vi "main.vi"() -> ()   [LabVIEW 2014]
uses:
  typedefs/ePathsAction.ctl
  typedefs/eMainAction.ctl
  typedefs/Alldata.ctl
  typedefs/NISTData.ctl
  typedefs/NIDataArray.ctl
  typedefs/NIData.ctl
  typedefs/PhasorRectangular.ctl
  typedefs/DUTData.ctl
  typedefs/NICalcAnalysis.ctl
  typedefs/CalcPhasorError.ctl
  typedefs/PlotDataArrays.ctl
  typedefs/PmuRawDataCluster.ctl
  typedefs/CalcAnalysis.ctl
  typedefs/ResultArray.ctl
  typedefs/Result.ctl
  typedefs/TVE_Fe_RFE.ctl
  <vilib>/Utility/file.llb/Write To Spreadsheet File (string).vi
panel:
  out "error out":errorcluster
  in  "btnSave":bool
  in  "btnMultiSrcAnalysis":bool
  in  "btnPlots":bool
  in  "Tab Control":T1(tab)
  out "Fluke Time":timestamp format="%^<%.3X\n%x>T"
  out "NIST Time":timestamp format="%^<%.3X\n%x>T"
  out "NIST VPhaseA Magnitude":cluster{"X":dbl, "Y":dbl}[](graph)
  out "Fluke VPhaseA Magnitude":cluster{"X":dbl, "Y":dbl}[](graph)
  out "NIST Meas - Fluke True TVE":string[][](table)
  out "NIST Meas - Fluke PMU TVE":string[][](table)
  out "CUT Results - CCS Results TVE":string[][](table)
  out "Results Table":string[][](table)
  in  "btnSrcAnalysis":bool
  in  "btnExit":bool
  in  "error in (no error)":errorcluster
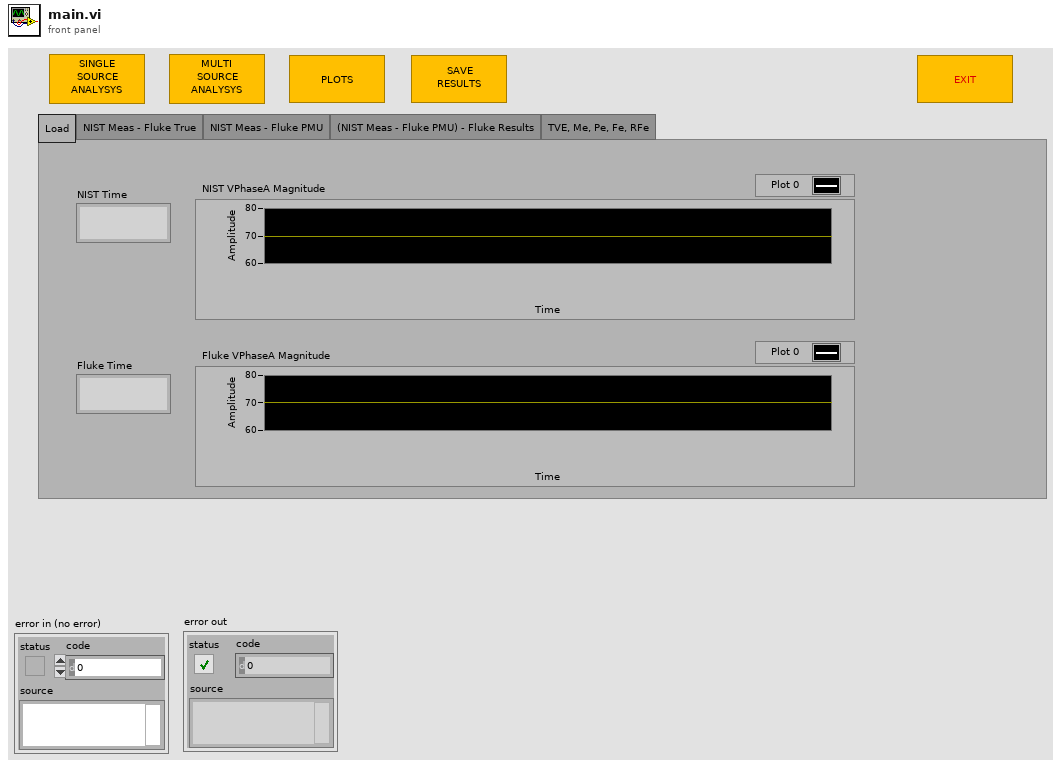
[diagram p1: front panel]
types:
  T1 = enum32{"Load", "NIST Meas - Fluke True", "NIST Meas - Fluke PMU", "(NIST Meas - Fluke PMU) - Fluke Results", "TVE, Me, Pe, Fe, RFe"}
  T2 = typedef "ResultArray.ctl" = T3[]
  T3 = typedef "Result.ctl" = cluster{"Time Stamp":timestamp, "VPhaseA":T4, "VPhaseB":T4, "VPhaseC":T4, "IPhaseA":T4, "IPhaseB":T4, "IPhaseC":T4}
  T4 = typedef "TVE_Fe_RFE.ctl" = cluster{"TVE":dbl, "Fe":dbl, "RFe":dbl}
  T5 = typedef "Alldata.ctl" = cluster{"NISTData":T6, "FlukeData":T13, "Params":dbl[]}
  T6 = typedef "NISTData.ctl" = cluster{"NIDataArray":T7, "DUTDataArray":T10[], "DataAnlysisArray":T11[]}
  T7 = typedef "NIDataArray.ctl" = T8[]
  T8 = typedef "NIData.ctl" = cluster{"Time":dbl, "VA":T9, "VB":T9, "VC":T9, "V+":T9, "IA":T9, "IB":T9, "IC":T9, "I+":T9, "Freq":dbl, "ROCOF":dbl, "TimeStamp":timestamp}
  T9 = typedef "PhasorRectangular.ctl" = cluster{"Real":dbl, "Imaginary":dbl}
  T10 = typedef "DUTData.ctl" = cluster{"Time":dbl, "VA":T9, "VB":T9, "VC":T9, "V1":T9, "IA":T9, "IB":T9, "IC":T9, "I1":T9, "Freq":dbl, "ROCOF":dbl, "TimeStamp":timestamp}
  T11 = typedef "NICalcAnalysis.ctl" = cluster{"Time":dbl, "VPhaseA":T12, "VPhaseB":T12, "VPhaseC":T12, "VPosSeq":T12, "IPhaseA":T12, "IPhaseB":T12, "IPhaseC":T12, "IPosSeq":T12, "Fe":dbl, "RFe":dbl, "TimeStamp":timestamp}
  T12 = typedef "CalcPhasorError.ctl" = cluster{"TVE":dbl, "MagErr":dbl, "PhaseErr":dbl}
  T13 = typedef "PlotDataArrays.ctl" = cluster{"PMUDataArray":T14[], "ModelDataArray":T14[], "DataAnalysisArray":T15[]}
  T14 = typedef "PmuRawDataCluster.ctl" = cluster{"TimeStamp":timestamp, "VPhaseA":T9, "VPhaseB":T9, "VPhaseC":T9, "VPosSeq":T9, "IPhaseA":T9, "IPhaseB":T9, "IPhaseC":T9, "IPosSeq":T9, "FREQUENCY":dbl, "ROCOF":sgl}
  T15 = typedef "CalcAnalysis.ctl" = cluster{"TimeStamp":timestamp, "VPhaseA":T12, "VPhaseB":T12, "VPhaseC":T12, "VPosSeq":T12, "IPhaseA":T12, "IPhaseB":T12, "IPhaseC":T12, "IPosSeq":T12, "Fe":dbl, "RFe":dbl}
  T16 = typedef "eMainAction.ctl" = enum16{"Init", "ProcessUI", "Exit"}
  T17 = typedef "ePathsAction.ctl" = enum16{"Set", "Get", "Load", "Save", "Default", "Exit"}
  T18 = enum32{"Load", "NIST Meas - Fluke True", "NIST Meas - Fluke PMU", "(NIST Meas - Fluke PMU) - Fluke Results"}
  T19 = typedef "Paths.ctl" = cluster{"BasePath":path, "CutPath":path, "LastCutPath":path, "CCSPath":path, "LastCCSPath":path, "ResultsPath":path}
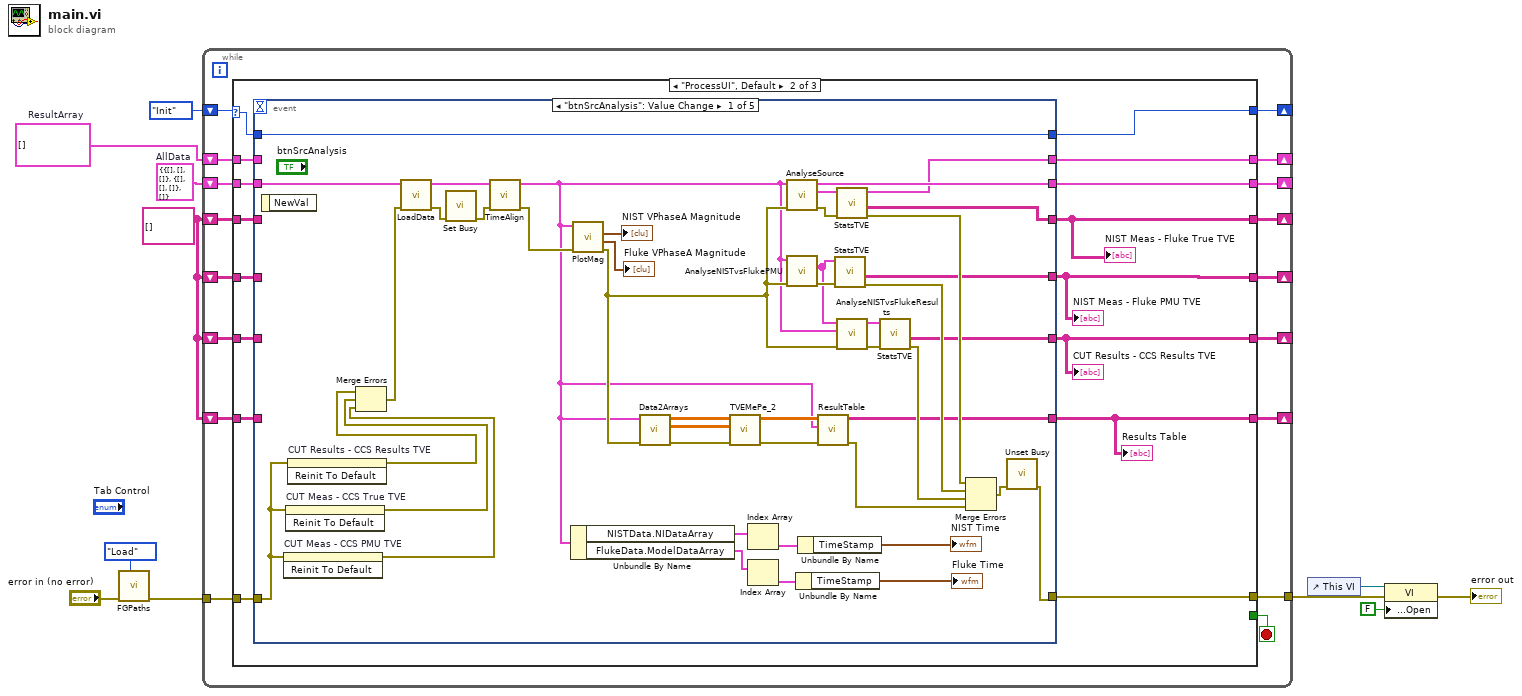
[diagram p0: block diagram]
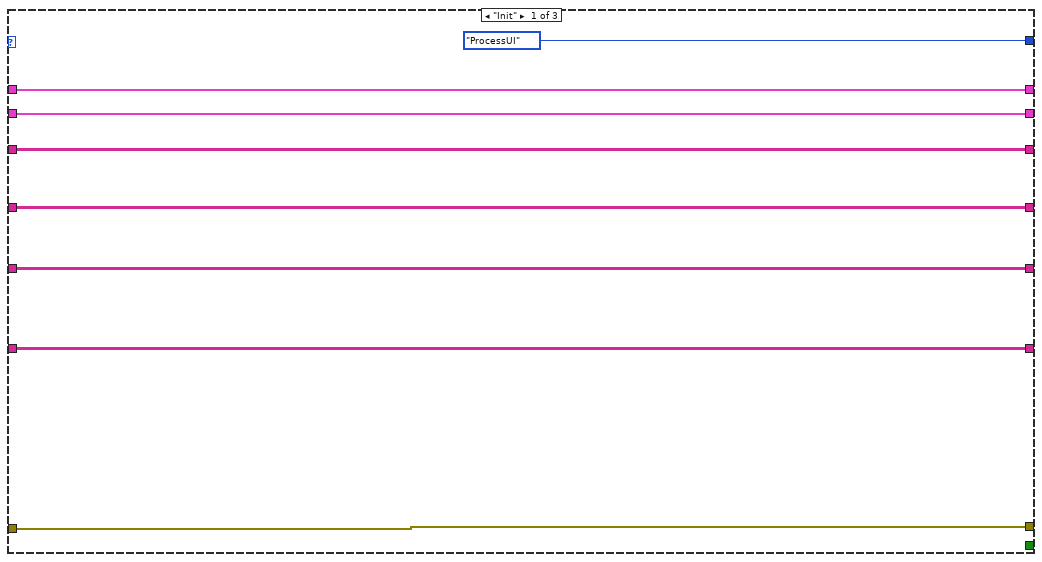
[diagram p2: hidden frame]
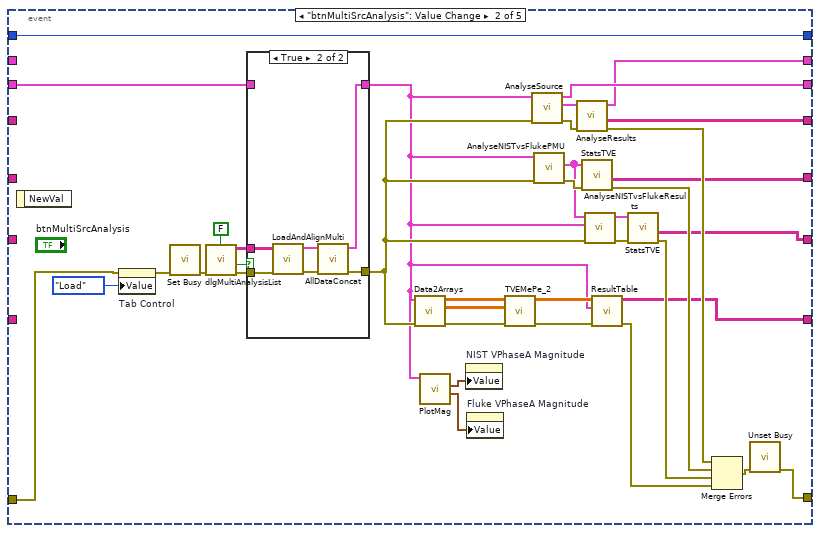
[diagram p3: hidden frame]
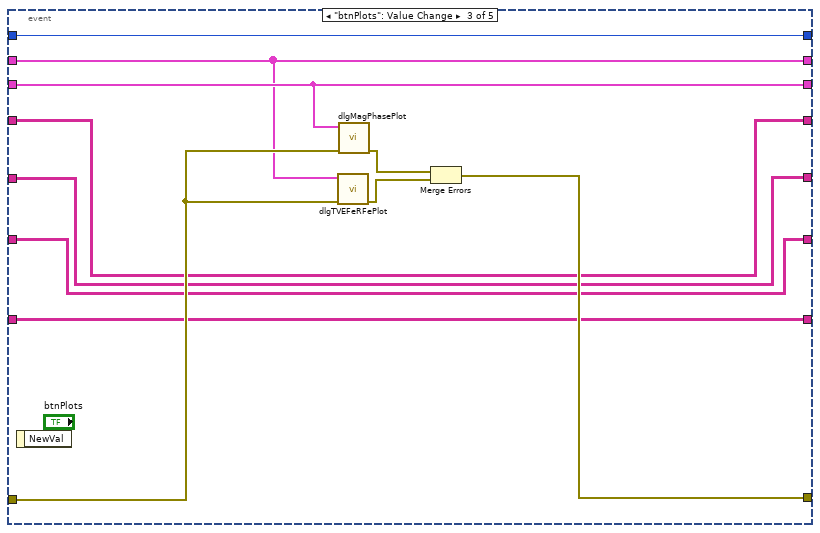
[diagram p5: hidden frame]
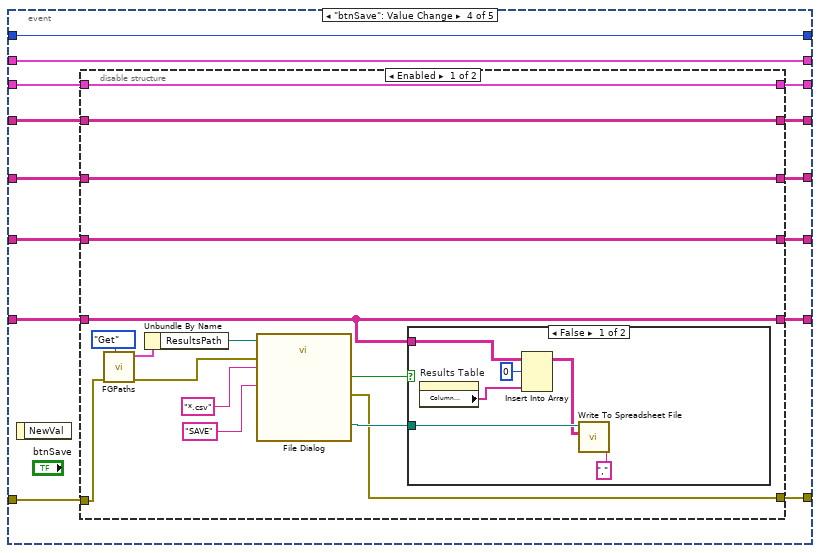
[diagram p6: hidden frame]
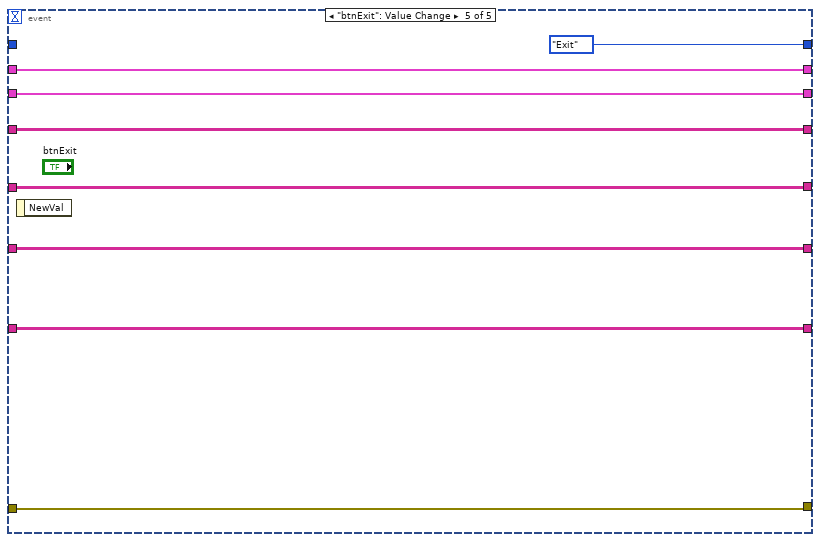
[diagram p9: hidden frame]
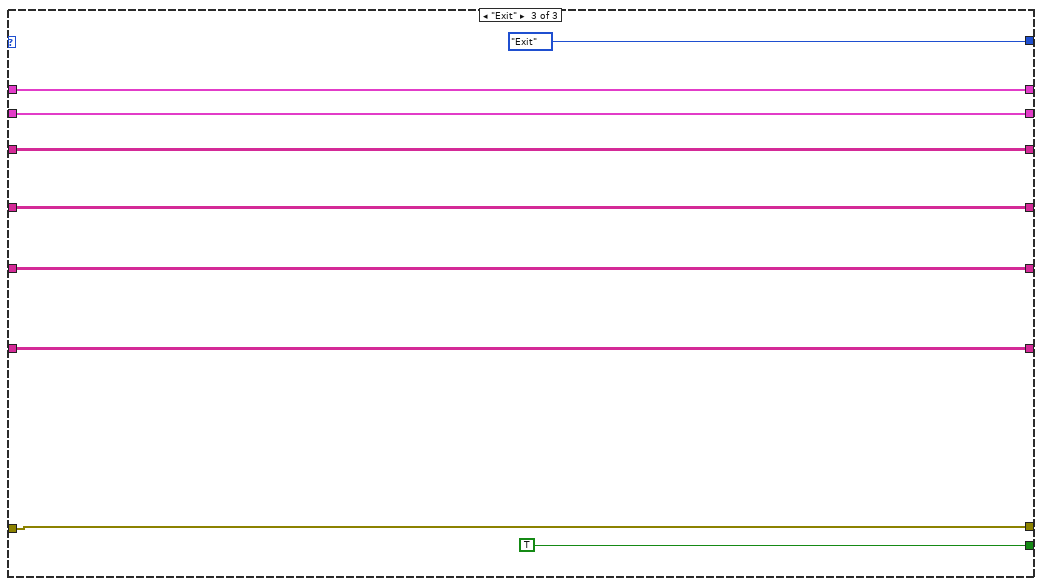
[diagram p10: hidden frame]
diagram:
  w2 = string[][] [] ("StringArray")
  w6 = T2 []  # ResultArray
  w7 = T5 {"NISTData"={"NIDataArray"=[], "DUTDataArray"=[], "DataAnlysisArray"=[]}, "FlukeData"={"PMUDataArray"=[], "ModelDataArray"=[], "DataAnalysisArray"=[]}, "Params"=[]}  # AllData
  n1 = call "FGPaths.vi"("ePathsAction"=ePathsAction."Load", "error in (no error)"="error in (no error)") -> ("error out"=w8:errorcluster)  [unwired: 8 in, 1 out]
  n2 = while {
    shift-right: [w27] -> _
    shift-left: eMainAction."Init" ("eMainAction") -> [w28]
    tunnel: w8 -> [w26]
    tunnel: [w25] -> w4
    shift-right: [w22] -> _
    shift-left: w7 -> [w23]
    shift-right: [w21] -> _
    shift-left: w6 -> [w20]
    shift-right: [w19] -> _
    shift-left: w2 -> [w18]
    shift-right: [w17] -> _
    shift-left: w2 -> [w16]
    shift-right: [w15] -> _
    shift-left: w2 -> [w14]
    shift-right: [w13] -> _
    shift-left: w2 -> [w12]
    stop <- w24 stop-if-true
    n3 = case shown="\"ProcessUI\", Default" w28 {
      selector: w28 -> [_ w49 _]
      tunnel: [eMainAction."ProcessUI" ("eMainAction") w50 eMainAction."Exit" ("eMainAction")] -> w27
      tunnel: w26 -> [w35 w52 w208]
      tunnel: [w35 w51 w208] -> w25
      tunnel: [_ _ TRUE] -> w24
      tunnel: [w34 w48 w206] -> w22
      tunnel: w23 -> [w34 w47 w206]
      tunnel: [w33 w46 w207] -> w21
      tunnel: w20 -> [w33 w45 w207]
      tunnel: [w32 w41 w205] -> w19
      tunnel: w18 -> [w32 w44 w205]
      tunnel: [w31 w43 w204] -> w17
      tunnel: w16 -> [w31 w42 w204]
      tunnel: [w30 w39 w203] -> w15
      tunnel: w14 -> [w30 w40 w203]
      tunnel: [w29 w38 w202] -> w13
      tunnel: w12 -> [w29 w37 w202]
      frame "Init" {
      }
      frame "ProcessUI", Default {
        n4 = event shown="[0] \"btnSrcAnalysis\": Value Change" {
          selector: _ -> [_ _ _ _ _]
          dyn-events: _ -> [_ _ _ _ _]
          timeout: _ -> [_ _ _ _ _]
          tunnel: [w88 w122 w147 w162 w197] -> w51
          tunnel: w52 -> [w66 w124 w151 w164 w197]
          tunnel: [w78 w121 w146 w166 eMainAction."Exit" ("eMainAction")] -> w50
          tunnel: w49 -> [w78 w121 w146 w166 _]
          tunnel: [w95 w128 w152 w160 w200] -> w48
          tunnel: w47 -> [w91 w129 w152 w161 w200]
          tunnel: [w94 w125 w150 w165 w199] -> w46
          tunnel: w45 -> [_ _ w150 w165 w199]
          tunnel: [w77 w120 w145 w155 w198] -> w41
          tunnel: w44 -> [_ _ w145 w163 w198]
          tunnel: [w72 w116 w144 w158 w196] -> w43
          tunnel: w42 -> [_ _ w144 w159 w196]
          tunnel: [w63 w109 w143 w156 w195] -> w39
          tunnel: w40 -> [_ _ w143 w157 w195]
          tunnel: [w55 w101 w142 w154 w194] -> w38
          tunnel: w37 -> [_ _ w142 w153 w194]
          event "btnSrcAnalysis": Value Change {
            n5 = event-data() -> ()  [unwired: 1 in, 1 out]
            n6 = invoke on="CUT Meas - CCS PMU TVE" class="Tbl (strict)" method="Reinit To Default"(error in=w66) -> (error out=w71:errorcluster)  [unwired: 2 in, 2 out]
            n7 = invoke on="CUT Meas - CCS True TVE" class="Tbl (strict)" method="Reinit To Default"(error in=w66) -> (error out=w70:errorcluster)  [unwired: 2 in, 2 out]
            n8 = invoke on="CUT Results - CCS Results TVE" class="Tbl (strict)" method="Reinit To Default"(error in=w66) -> (error out=w68:errorcluster)  [unwired: 2 in, 2 out]
            n9 = Merge Errors(w68, w70, w71) -> (w69:errorcluster)
            n10 = call "LoadData.vi"("error in (no error)"=w69, "AllData In"=w91) -> ("error out"=w90:errorcluster, "AllData Out"=w92:T5)  [unwired: 8 in]
            n11 = call <vilib>:"Set Busy.vi"("error in (no error)"=w90) -> ("error out"=w89:errorcluster)  [unwired: 9 in, 1 out]
            n12 = call "TimeAlign.vi"("error in (no error)"=w89, "AllData In"=w92) -> ("error out"=w87:errorcluster, "AllData Out"=w54:T5)  [unwired: 8 in]
            n13 = Unbundle By Name(w54) -> ("NISTData.NIDataArray"=w84:T7, "FlukeData.ModelDataArray"=w83:T14[])
            n14 = call "PlotMag.vi"("error in (no error)"=w87, "AllData In"=w54) -> ("error out"=w58:errorcluster, "NistPlot"=→"Fluke VPhaseA Magnitude":cluster{"X":dbl, "Y":dbl}[], "FlukePlot"=→"NIST VPhaseA Magnitude":cluster{"X":dbl, "Y":dbl}[])  [unwired: 7 in]
            n15 = call "Data2Arrays.vi"("error in (no error)"=w58, "AllData"=w54) -> ("error out"=w57:errorcluster, "Fluke"=w60:dbl[][], "NIST"=w61:dbl[][])  [unwired: 7 in]
            n16 = call "TVEMePe_2.vi"("error in (no error)"=w57, "Fluke"=w60, "NIST"=w61) -> ("error out"=w56:errorcluster, "TVEMePe"=w59:dbl[][])  [unwired: 7 in]
            n17 = Index Array(array=w84) -> (element=w82:T8)  [unwired: 1 in]
            n18 = Index Array(array=w83) -> (element=w81:T14)  [unwired: 1 in]
            n19 = call "AnalyseSource.vi"("error in (no error)"=w58, "AllData In"=w54) -> ("error out"=w93:errorcluster, "ResultArray"=w96:T2, "AllData Out"=w95:T5)  [unwired: 7 in]
            n20 = call "AnalyseNISTvsFlukePMU.vi"("error in (no error)"=w58, "AllData In"=w54) -> ("error out"=w76:errorcluster, "ResultArray"=w67:T2)  [unwired: 7 in, 1 out]
            n21 = Unbundle By Name(w81) -> ("TimeStamp"=→"Fluke Time":timestamp)
            n22 = Unbundle By Name(w82) -> ("TimeStamp"=→"NIST Time":timestamp)
            n23 = call "ResultTable.vi"("error in (no error)"=w56, "AllData"=w54, "TVEMePe"=w59) -> ("error out"=w53:errorcluster, "Results Table"=w55:string[][])  [unwired: 7 in]
            n24 = call "StatsTVE.vi"("error in (no error)"=w76, "ResultArrayIn"=w67) -> ("error out"=w73:errorcluster, "StringArray"=w72:string[][])  [unwired: 6 in, 2 out]
            n25 = call "StatsTVE.vi"("error in (no error)"=w93, "ResultArrayIn"=w96) -> ("error out"=w74:errorcluster, "StringArray"=w77:string[][], "ResultArrayOut"=w94:T2)  [unwired: 6 in, 1 out]
            n26 = call "AnalyseNISTvsFlukeResults.vi"("error in (no error)"=w58, "AllData In"=w54, "NISTResults"=w67) -> ("error out"=w65:errorcluster, "Resultarray"=w64:T3[])  [unwired: 7 in]
            n27 = call "StatsTVE.vi"("error in (no error)"=w65, "ResultArrayIn"=w64) -> ("error out"=w62:errorcluster, "StringArray"=w63:string[][])  [unwired: 6 in, 2 out]
            n28 = Merge Errors(w74, w73, w62, w53) -> (w75:errorcluster)
            n29 = call <vilib>:"Unset Busy.vi"("error in (no error)"=w75) -> ("error out"=w88:errorcluster)  [unwired: 10 in]
          }
          event "btnMultiSrcAnalysis": Value Change {
            n30 = event-data() -> ()  [unwired: 1 in, 1 out]
            n31 = property on="Tab Control" class="TabCtl (strict)"(error in=w124, "Value"=T18."Load" ("Tab Control")) -> (error out=w97:errorcluster)  [unwired: 1 in, 1 out]
            n32 = call <vilib>:"Set Busy.vi"("error in (no error)"=w97) -> ("error out"=w123:errorcluster)  [unwired: 9 in, 1 out]
            n33 = call "dlgMultiAnalysisList.vi"("StandAlone (true)"=FALSE, "error in (no error)"=w123) -> ("error out"=w131:errorcluster, "Analyse"=w132:bool, "FileList"=w130:string[][])  [unwired: 7 in]
            n34 = case shown="True" w132 {
              tunnel: w131 -> [w135 w140]
              tunnel: [w135 w136] -> w102
              tunnel: w130 -> [_ w141]
              tunnel: [w134 w138] -> w98
              tunnel: w129 -> [w134 _]
              frame False {
              }
              frame True {
                n35 = call "LoadAndAlignMulti.vi"("error in (no error)"=w140, "FileList"=w141) -> ("error out"=w137:errorcluster, "AllDataArray"=w139:T5[])  [unwired: 8 in]
                n36 = call "AllDataConcat.vi"("error in (no error)"=w137, "AllDataArray"=w139) -> ("error out"=w136:errorcluster, "AllData"=w138:T5)  [unwired: 8 in]
              }
            }
            n37 = call "Data2Arrays.vi"("error in (no error)"=w102, "AllData"=w98) -> ("error out"=w105:errorcluster, "Fluke"=w107:dbl[][], "NIST"=w108:dbl[][])  [unwired: 7 in]
            n38 = call "PlotMag.vi"("AllData In"=w98) -> ("NistPlot"=w100:cluster{"X":dbl, "Y":dbl}[], "FlukePlot"=w99:cluster{"X":dbl, "Y":dbl}[])  [unwired: 8 in, 1 out]
            n39 = property on="NIST VPhaseA Magnitude" class="XYGraph (strict)"("Value"=w99) -> ()  [unwired: 2 in, 2 out]
            n40 = property on="Fluke VPhaseA Magnitude" class="XYGraph (strict)"("Value"=w100) -> ()  [unwired: 2 in, 2 out]
            n41 = call "TVEMePe_2.vi"("error in (no error)"=w105, "Fluke"=w107, "NIST"=w108) -> ("error out"=w104:errorcluster, "TVEMePe"=w106:dbl[][])  [unwired: 7 in]
            n42 = call "AnalyseSource.vi"("error in (no error)"=w102, "AllData In"=w98) -> ("error out"=w126:errorcluster, "ResultArray"=w127:T2, "AllData Out"=w128:T5)  [unwired: 7 in]
            n43 = call "AnalyseNISTvsFlukePMU.vi"("error in (no error)"=w102, "AllData In"=w98) -> ("error out"=w117:errorcluster, "ResultArray"=w111:T2)  [unwired: 7 in, 1 out]
            n44 = call "AnalyseResults.vi"("error in (no error)"=w126, "ResultArrayIn"=w127) -> ("error out"=w118:errorcluster, "StringArray"=w120:string[][], "ResultArrayOut"=w125:T2)  [unwired: 6 in, 1 out]
            n45 = call "StatsTVE.vi"("error in (no error)"=w117, "ResultArrayIn"=w111) -> ("error out"=w115:errorcluster, "StringArray"=w116:string[][])  [unwired: 6 in, 2 out]
            n46 = call "AnalyseNISTvsFlukeResults.vi"("error in (no error)"=w102, "AllData In"=w98, "NISTResults"=w111) -> ("error out"=w113:errorcluster, "Resultarray"=w112:T3[])  [unwired: 7 in]
            n47 = call "ResultTable.vi"("error in (no error)"=w104, "AllData"=w98, "TVEMePe"=w106) -> ("error out"=w103:errorcluster, "Results Table"=w101:string[][])  [unwired: 7 in]
            n48 = call "StatsTVE.vi"("error in (no error)"=w113, "ResultArrayIn"=w112) -> ("error out"=w110:errorcluster, "StringArray"=w109:string[][])  [unwired: 6 in, 2 out]
            n49 = Merge Errors(w118, w115, w110, w103) -> (w119:errorcluster)
            n50 = call <vilib>:"Unset Busy.vi"("error in (no error)"=w119) -> ("error out"=w122:errorcluster)  [unwired: 10 in]
          }
          event "btnPlots": Value Change {
            n51 = event-data() -> ()  [unwired: 1 in, 1 out]
            n52 = call "dlgTVEFeRFePlot.vi"("error in (no error)"=w151, "ResultArray"=w150) -> ("error out"=w149:errorcluster)  [unwired: 9 in]
            n53 = call "dlgMagPhasePlot.vi"("error in (no error)"=w151, "AllData"=w152) -> ("error out"=w148:errorcluster)  [unwired: 9 in]
            n54 = Merge Errors(w148, w149) -> (w147:errorcluster)
          }
          event "btnSave": Value Change {
            n55 = event-data() -> ()  [unwired: 1 in, 1 out]
            n56 = disable-structure shown="Enabled" {
              disable-tunnel: w164 -> [w180 w189]
              disable-tunnel: w163 -> [w168 w193]
              disable-tunnel: [w176 w189] -> w162
              disable-tunnel: w161 -> [w171 w190]
              disable-tunnel: [w171 w190] -> w160
              disable-tunnel: w159 -> [w170 w192]
              disable-tunnel: [w170 w192] -> w158
              disable-tunnel: w157 -> [w169 w191]
              disable-tunnel: [w169 w191] -> w156
              disable-tunnel: [w168 w193] -> w155
              disable-tunnel: [w167 w188] -> w154
              disable-tunnel: w153 -> [w167 w188]
              frame Enabled {
                n57 = call "FGPaths.vi"("ePathsAction"=ePathsAction."Get", "error in (no error)"=w180) -> ("error out"=w177:errorcluster, "PathsOut"=w179:T19)  [unwired: 8 in]
                n58 = Unbundle By Name(w179) -> ("ResultsPath"=w175:path)
                n59 = call "File Dialog"("start path"=w175, "button label"="SAVE", "error in"=w177, "pattern (all files)"="*.csv") -> ("selected path"=w178:path, "cancelled"=w172:bool, "error out"=w176:errorcluster)  [unwired: 8 in, 1 out]
                n60 = case shown="False" w172 {
                  tunnel: w167 -> [w185 _]
                  tunnel: w178 -> [w186 _]
                  frame False {
                    n61 = property on="Results Table" class="Tbl (strict)"() -> ("Column Headers[]"=w182:string[])  [unwired: 2 in, 2 out]
                    n62 = Insert Into Array(array=w185, index (row)=0, new element=w182) -> (w183:string[][])  [unwired: 1 in]
                    n63 = call-poly <vilib>:"Write To Spreadsheet File.vi"("delimiter (\\t)"="," ("delimiter (\\t)"), "2D data"=w183, "file path (dialog if empty)"=w186) -> ()  [unwired: 5 in, 1 out]
                  }
                  frame True {
                  }
                }
              }
              frame Disabled {
              }
            }
          }
          event "btnExit": Value Change {
            n64 = event-data() -> ()  [unwired: 1 in, 1 out]
          }
        }
        "NIST Meas - Fluke PMU TVE" <- w43
        "NIST Meas - Fluke True TVE" <- w41
        "CUT Results - CCS Results TVE" <- w39
        "Results Table" <- w38
      }
      frame "Exit" {
      }
    }
  }
  n65 = control-ref of="This VI"() -> (w5:refnum<vi>)
  n66 = property class="VI"(reference=w5, error in=w4, "Front Panel.Open"=FALSE ("Front Panel Window:Open")) -> (error out=→"error out":errorcluster)  [unwired: 1 out]
